vi "XML to Populated Entry.vi"(1 "XML Data":string, 2 "Name":string) -> (0 "Experiment Data":T1)   [LabVIEW 2013]
uses:
  Types/Experiment Data.ctl
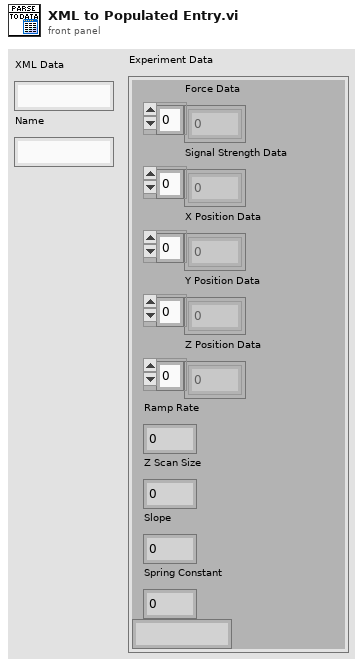
[diagram p1: front panel]
types:
  T1 = typedef "Experiment Data.ctl" = cluster{"Force Data":dbl[], "Signal Strength Data":dbl[], "X Position Data":dbl[], "Y Position Data":dbl[], "Z Position Data":dbl[], "Ramp Rate":dbl, "Z Scan Size":dbl, "Slope":dbl, "Spring Constant":dbl, "Version":string}
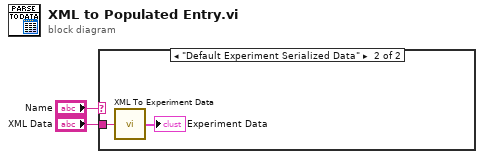
[diagram p0: block diagram]
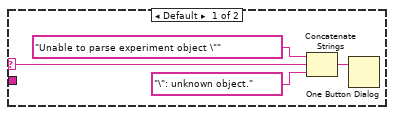
[diagram p2: hidden frame]
diagram:
  n1 = case shown="\"Default Experiment Serialized Data\"" "Name" {
    selector: "Name" -> [w4 _]
    tunnel: "XML Data" -> [_ w8]
    frame Default {
      n2 = Concatenate Strings("Unable to parse experiment object \"" ("string"), w4, "\": unknown object." ("string")) -> (w5:string)
      n3 = One Button Dialog(message=w5) -> ()  [unwired: 1 in, 1 out]
    }
    frame "Default Experiment Serialized Data" {
      n4 = call "XML To Experiment Data.vi"("XML Data"=w8) -> ("Experiment Data"=→"Experiment Data":T1)
    }
  }
